vi "Act_LabView_2p2_Team205.vi"() -> ()   [LabVIEW 2016]
uses:
  <vilib>/express/express arith-compare/Formula/XNode/ExpressFormulaBlockNode.xnode
panel:
  in  "c":dbl
  in  "b":dbl
  in  "a":dbl
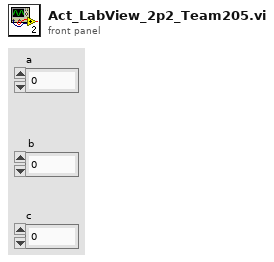
[diagram p1: front panel]
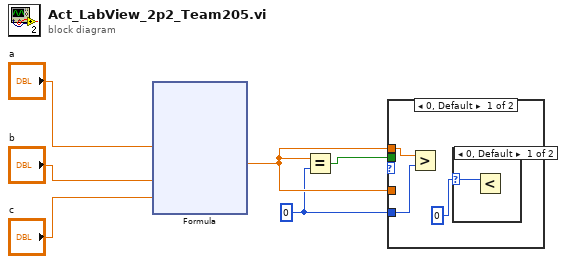
[diagram p0: block diagram]
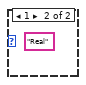
[diagram p2: hidden frame]
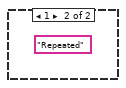
[diagram p3: hidden frame]
diagram:
  w1 = 0
  n1 = xnode "Formula"("a"="a", "b"="b", "c"="c") -> ("Result"=w2:dbl)  [unwired: 1 in, 1 out]
  n2 = Equal?(x=w2, y=w1) -> (x = y?=w3:bool)
  n3 = case shown="0, Default" {
    selector: _ -> [_ _]
    tunnel: w3 -> [_ _]
    tunnel: w2 -> [w9 _]
    tunnel: w2 -> [_ _]
    tunnel: w1 -> [w8 _]
    frame 0, Default {
      n4 = Greater?(x=w9, y=w8) -> ()  [unwired: 1 out]
      n5 = case shown="0, Default" 0 {
        selector: 0 -> [w10 _]
        frame 0, Default {
          n6 = Less?(x=w10) -> ()  [unwired: 1 in, 1 out]
        }
        frame 1 {
          (unwired) "Real"
        }
      }
    }
    frame 1 {
      (unwired) "Repeated"
    }
  }
